vi "Shooter Controller.vi"(8 "error in":errorcluster) -> ()   [LabVIEW 2019]
uses:
  <vilib>/Rock Robotics/WPI/Framework/Completion Status.ctl
  Shooter Setpoints.ctl
  Shooter Operations.ctl
  <vilib>/Rock Robotics/WPI/ThirdParty/REV Robotics/SPARK MAX/Typedef/Spark MAX Idle Mode.ctl
  <vilib>/Rock Robotics/WPI/ThirdParty/REV Robotics/SPARK MAX/Typedef/Spark MAX Control Type.ctl
  <vilib>/Rock Robotics/Network Tables/NT Write Number.vi
  <vilib>/Rock Robotics/Network Tables/NT Read Number.vi
  Framework/Robot Global Data.vi
  28b4446c-53d7-42fe-a716-59488cbe5fc2.vi
  <vilib>/Rock Robotics/Network Tables/NT Write Boolean.vi
panel:
  in  "Flang Setpoint 2":dbl=0.5
  in  "Transfer Setpoint 2":dbl=0.3
  out "shooter 2":dbl(graph)
  out "Waveform Chart 2":dbl(graph)
  out "Waveform Chart":dbl(graph)
  in  "Transfer Setpoint":dbl=0.3
  out "shooter":dbl(graph)
  in  "Flang Setpoint":dbl=0.5
  in  "override":bool=TRUE
  in  "Manual Flywheel":dbl(slide)
  in  "Current Limit A (100)":sgl=100.0
  in  "turret pid":T1={"P Gain"=0.07, "I Gain"=0.0002, "D Gain"=0.0, "F Gain"=0.0, "I Zone"=2.0, "Min Output"=-1.0, "Max Output"=1.0}
  in  "hood pid":T1={"P Gain"=0.1, "I Gain"=0.0002, "D Gain"=0.0, "F Gain"=0.0, "I Zone"=2.0, "Min Output"=-1.0, "Max Output"=1.0}
  in  "flywheel pid":T1={"P Gain"=0.001, "I Gain"=0.0, "D Gain"=0.0, "F Gain"=0.000185, "I Zone"=100.0, "Min Output"=0.0, "Max Output"=1.0}
  in  "Interactive Values":T2
  out "Current\nCmd":string
  in  "Buttons":cluster{"Execute Cmd":bool, "Abort Cmd":bool}
  out "Command Timing":cluster{"Start Time (ms)":u32, "Iterations":i32}
  out "Status":T4
  # "Tip: It may be helpful to observe inputs and sensor values.\nYou may also want to display tuning or debugging controls."
  # "Interactive Command: You may fill in the settings for a command\nand schedule it with the Execute button. You can observe and abort\nany command while fine tuning the code for the controller."
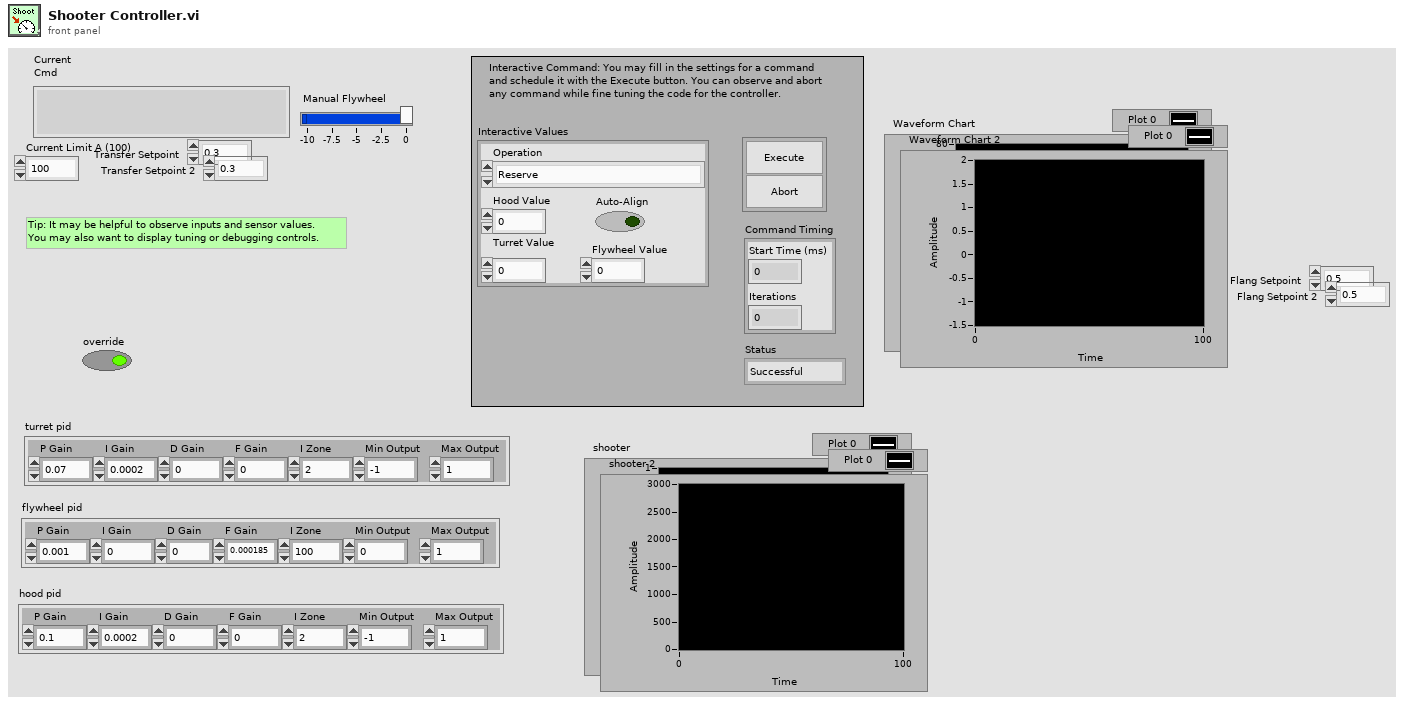
[diagram p1: front panel]
types:
  T1 = cluster{"P Gain":dbl, "I Gain":dbl, "D Gain":dbl, "F Gain":dbl, "I Zone":dbl, "Min Output":dbl, "Max Output":dbl}
  T2 = typedef "Shooter Setpoints.ctl" = cluster{"Operation":T3, "Hood Value":dbl, "Flywheel Value":dbl, "Turret Value":dbl, "Auto-Align":bool}
  T3 = typedef "Shooter Operations.ctl" = enum16{"Reserve", "Read Current", "Immediate", "Shoot", "Reverse Flywheel", "Shoot until no balls"}
  T4 = typedef "Completion Status.ctl" = enum16{"Successful", "Aborted", "Incomplete"}
  T5 = typedef "Spark MAX Idle Mode.ctl" = enum16{"Coast", "Brake"}
  T6 = typedef "WPI_MotorControlDeviceRef.ctl" = cluster{"DeviceStatus":errorcluster, "Type":T7, "PWM":cluster{"PWM Channel":T8, "DeadBand":T9}, "CAN":cluster{"Device Number":u8, "SetOutput VI Ref":variant, "GetOutput VI Ref":variant, "Enable VI Ref":variant, "Disable VI Ref":variant, "Data":variant}, "Invert":bool, "DIO PWM":cluster{"PWM \"Enable\" Channel":T8, "DIOChannel":T10, "PWM Rate":dbl}}
  T7 = typedef "WPI_MotorControlType.ctl" = enum16{"PWM", "CAN", "DIO PWM"}
  T8 = typedef "FPGA_DIOPWMChannel.ctl" = enum8{"PWM 0", "PWM 1", "PWM 2", "PWM 3", "PWM 4", "PWM 5", "PWM 6", "PWM 7", "PWM 8", "PWM 9", "PWM MXP 0", "PWM MXP 1", "PWM MXP 2", "PWM MXP 3", "PWM MXP 4", "PWM MXP 5", "PWM MXP 6", "PWM MXP 7", "PWM MXP 8", "PWM MXP 9", "Invalid"}
  T9 = typedef "WPI_PWMDeadband.ctl" = cluster{"Name":string, "maxPositivePwm":i32, "minPositivePwm":i32, "centerPwm":i32, "maxNegativePwm":i32, "minNegativePwm":i32, "angularRange":u16}
  T10 = typedef "FPGA_DIOChannel.ctl" = enum8{"DIO 0", "DIO 1", "DIO 2", "DIO 3", "DIO 4", "DIO 5", "DIO 6", "DIO 7", "DIO 8", "DIO 9", "DIO MXP 0", "DIO MXP 1", "DIO MXP 2", "DIO MXP 3", "DIO MXP 4", "DIO MXP 5", "DIO MXP 6", "DIO MXP 7", "DIO MXP 8", "DIO MXP 9", "DIO MXP 10", "DIO MXP 11", "DIO MXP 12", "DIO MXP 13", "DIO MXP 14", "DIO MXP 15", "SPI Port CS1", "SPI Port CS2", "SPI Port CS3", "SPI Port MISO", "SPI Port MOSI", "Invalid"}
  T11 = typedef "Command Status Info.ctl" = cluster{"Name":string, "Status":T4, "notifier out":T12}
  T12 = typedef "Completion Notifier.ctl" = refnum<notifier>
  T13 = cluster{"Current Command":T2, "Command Timing":cluster{"Start Time (ms)":u32, "Iterations":i32}, "Command Arguments":cluster{"Command Info":T11, "Description":string, "Default Command":T2, "queue out":refnum<queue>, "Subsystem Name":string}}
  T14 = typedef "Spark MAX Control Type.ctl" = enum16{"Percent VBus", "Voltage", "Velocity", "Position", "Smart Motion", "Current", "Smart Velocity"}
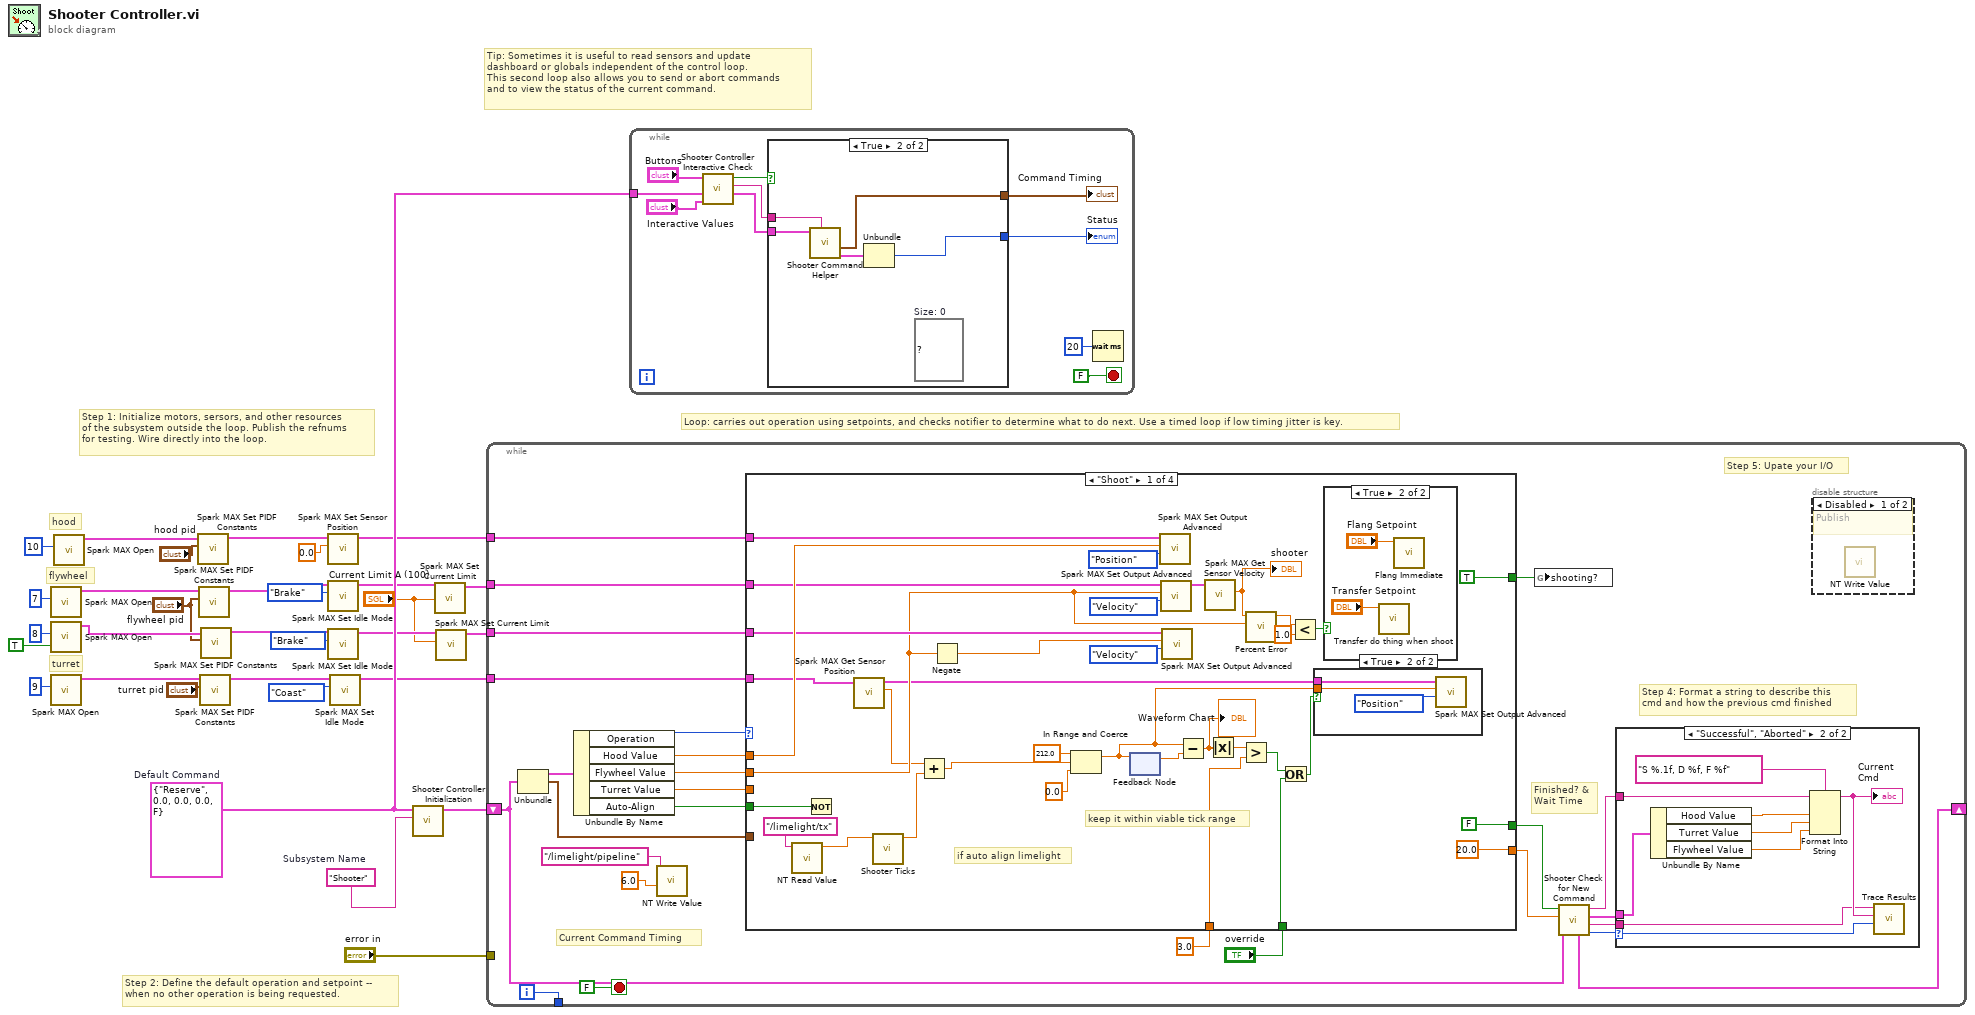
[diagram p0: block diagram]
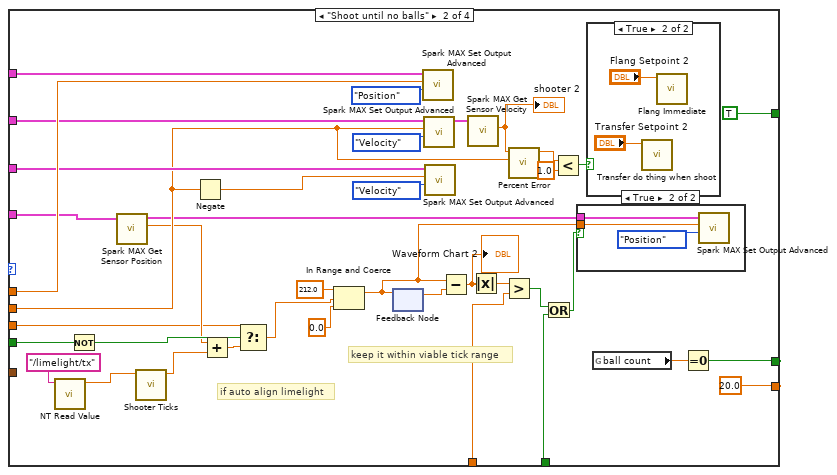
[diagram p6: hidden frame]
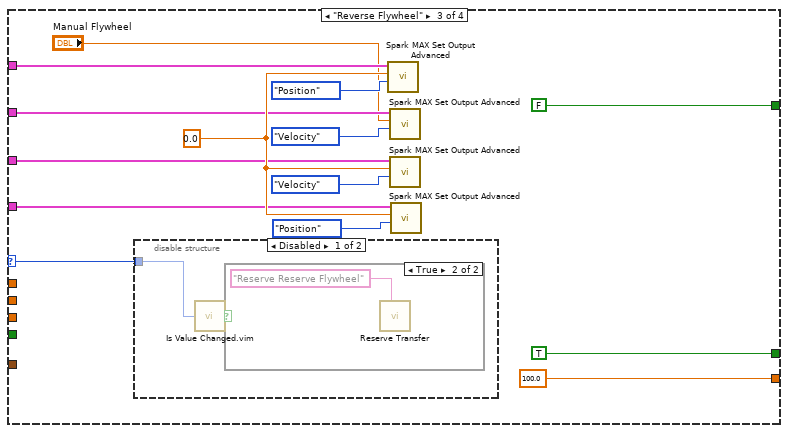
[diagram p9: hidden frame]
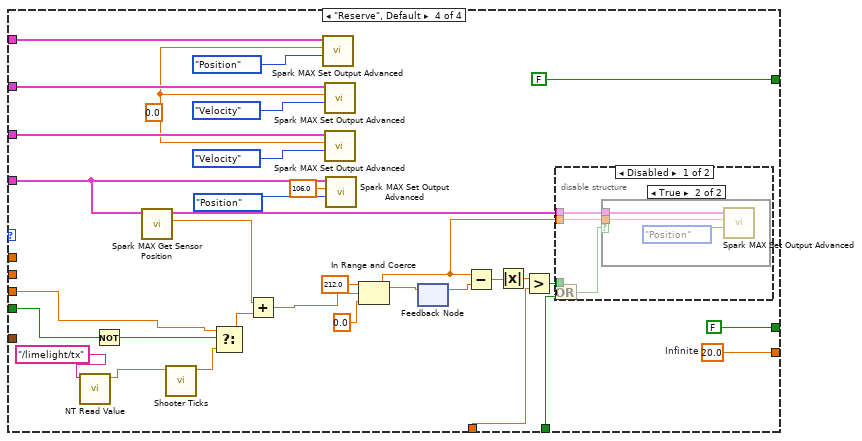
[diagram p12: hidden frame]
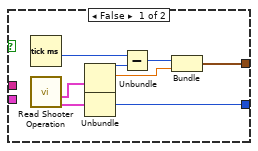
[diagram p15: hidden frame]
diagram:
  w28 = T2 {"Operation"=enum."Reserve", "Hood Value"=0.0, "Flywheel Value"=0.0, "Turret Value"=0.0, "Auto-Align"=FALSE}  # Default Command
  w29 = "Shooter"  # Subsystem Name
  # "turret"
  # "flywheel"
  # "hood"
  # "Tip: Sometimes it is useful to read sensors and update\ndashboard or globals independent of the control loop.\nThis second loop also allows you to send or abort commands\nand to view the status of the current command."
  # "Step 2: Define the default operation and setpoint --\nwhen no other operation is being requested."
  # "Step 1: Initialize motors, sersors, and other resources\nof the subsystem outside the loop. Publish the refnums\nfor testing. Wire directly into the loop."
  # "Loop: carries out operation using setpoints, and checks notifier to determine what to do next. Use a timed loop if low timing jitter is key."
  n1 = call <vilib>:"Spark MAX Open.vi"("Device Number"=u8 7) -> ("MotorControlDeviceRef"=w16:T6)  [unwired: 9 in, 1 out]
  n2 = call <vilib>:"Spark MAX Open.vi"("Invert"=TRUE, "Device Number"=u8 8) -> ("MotorControlDeviceRef"=w15:T6)  [unwired: 8 in, 1 out]
  n3 = call <vilib>:"Spark MAX Open.vi"("Device Number"=u8 9) -> ("MotorControlDeviceRef"=w14:T6)  [unwired: 9 in, 1 out]
  n4 = call <vilib>:"Spark MAX Open.vi"("Device Number"=u8 10) -> ("MotorControlDeviceRef"=w21:T6)  [unwired: 9 in, 1 out]
  n5 = call <vilib>:"Spark MAX Set PIDF Constants.vi"("PID Constants"="hood pid", "MotorControlDeviceRef"=w21) -> ("MotorControlDeviceRef"=w20:T6)  [unwired: 8 in, 1 out]
  n6 = call <vilib>:"Spark MAX Set PIDF Constants.vi"("PID Constants"="flywheel pid", "MotorControlDeviceRef"=w16) -> ("MotorControlDeviceRef"=w11:T6)  [unwired: 8 in, 1 out]
  n7 = call <vilib>:"Spark MAX Set PIDF Constants.vi"("PID Constants"="turret pid", "MotorControlDeviceRef"=w14) -> ("MotorControlDeviceRef"=w8:T6)  [unwired: 8 in, 1 out]
  n8 = call <vilib>:"Spark MAX Set PIDF Constants.vi"("PID Constants"="flywheel pid", "MotorControlDeviceRef"=w15) -> ("MotorControlDeviceRef"=w12:T6)  [unwired: 8 in, 1 out]
  n9 = call <vilib>:"Spark MAX Set Sensor Position.vi"("Position"=0.0, "MotorControlDeviceRef"=w20) -> ("MotorControlDeviceRef"=w18:T6)  [unwired: 8 in, 1 out]
  n10 = call <vilib>:"Spark MAX Set Idle Mode.vi"("Idle Mode"=Spark_MAX_Idle_Mode."Brake", "MotorControlDeviceRef in"=w11) -> ("MotorControlDeviceRef out"=w6:T6)  [unwired: 8 in, 1 out]
  n11 = call <vilib>:"Spark MAX Set Idle Mode.vi"("Idle Mode"=Spark_MAX_Idle_Mode."Brake", "MotorControlDeviceRef in"=w12) -> ("MotorControlDeviceRef out"=w4:T6)  [unwired: 8 in, 1 out]
  n12 = call <vilib>:"Spark MAX Set Idle Mode.vi"("Idle Mode"=Spark_MAX_Idle_Mode."Coast", "MotorControlDeviceRef in"=w8) -> ("MotorControlDeviceRef out"=w1:T6)  [unwired: 8 in, 1 out]
  n13 = call "Shooter Controller Initialization.vi"("Subsystem Name"=w29, "Default Command"=w28) -> ("Current Command"=w30:T13)  [unwired: 9 in]
  n14 = call <vilib>:"Spark MAX Set Current Limit.vi"("Current Limit A (100)"="Current Limit A (100)", "MotorControlDeviceRef in"=w6) -> ("MotorControlDeviceRef out"=w5:T6)  [unwired: 8 in, 1 out]
  n15 = call <vilib>:"Spark MAX Set Current Limit.vi"("Current Limit A (100)"="Current Limit A (100)", "MotorControlDeviceRef in"=w4) -> ("MotorControlDeviceRef out"=w3:T6)  [unwired: 8 in, 1 out]
  n16 = while {
    shift-right: [w53] -> _
    shift-left: w30 -> [w46]
    tunnel: [w56] -> _
    tunnel: "error in" -> [_]
    tunnel: w18 -> [w45]
    tunnel: w5 -> [w44]
    tunnel: w1 -> [w43]
    tunnel: w3 -> [w39]
    i -> [w56]
    stop <- FALSE stop-if-true
    # "Step 5: Upate your I/O"
    # "Step 4: Format a string to describe this\ncmd and how the previous cmd finished"
    # "Current Command Timing"
    # "Finished? &\nWait Time"
    n17 = Unbundle(w46) -> ("Current Command"=w55:T2, "Command Timing"=w54:cluster{"Start Time (ms)":u32, "Iterations":i32})  [unwired: 1 out]
    n18 = Unbundle By Name(w55) -> ("Operation"=w37:T3, "Hood Value"=w40:dbl, "Flywheel Value"=w42:dbl, "Turret Value"=w41:dbl, "Auto-Align"=w32:bool)
    n19 = call-poly <vilib>:"NT Write Value.vi"("Numeric"=6.0, "Name"="/limelight/pipeline") -> ()  [unwired: 9 in, 1 out]
    n20 = case shown="\"Shoot\"" w37 {
      selector: w37 -> [_ _ w151 _]
      tunnel: [20.0 ("Infinite") 20.0 ("Infinite") 100.0 ("Infinite") w199] -> w51
      tunnel: [FALSE ("ignore previous (F)") w111 TRUE ("ignore previous (F)") FALSE ("ignore previous (F)")] -> w52
      tunnel: w54 -> [_ _ _ _]
      tunnel: w45 -> [w99 w144 w159 w196]
      tunnel: w44 -> [w88 w132 w158 w193]
      tunnel: w43 -> [w81 w125 w156 w186]
      tunnel: w40 -> [w98 w143 _ _]
      tunnel: w42 -> [w85 w129 _ _]
      tunnel: w41 -> [_ w108 _ w183]
      tunnel: w32 -> [w97 w142 _ w185]
      tunnel: w39 -> [w87 w131 w157 w191]
      tunnel: [TRUE ("shooting?") TRUE ("shooting?") FALSE ("shooting?") FALSE ("shooting?")] -> w38
      tunnel: "override" -> [w72 w116 _ w172]
      tunnel: 3.0 ("y") -> [w71 w115 _ w174]
      frame "Shoot" {
        # "keep it within viable tick range"
        # "if auto align limelight"
        n21 = call-poly <vilib>:"NT Read Value.vi"("Name"="/limelight/tx") -> ("Numeric"=w69:dbl)  [unwired: 9 in, 1 out]
        n22 = Not(x=w97) -> ()  [unwired: 1 out]
        n23 = call <vilib>:"Spark MAX Get Sensor Position.vi"("MotorControlDevRef in"=w81) -> ("Sensor Position"=w79:dbl, "MotorControlDevRef out"=w80:T6)  [unwired: 7 in, 2 out]
        n24 = call "Shooter Ticks.vi"("limelight"=w69) -> ("ticks"=w68:dbl)  [unwired: 10 in]
        n25 = Add(x=w79, y=w68) -> (x+y=w67:dbl)
        n26 = Negate(x=w85) -> (-x=w90:dbl)
        n27 = In Range and Coerce(upper limit=212.0, x=w67, lower limit=0.0) -> (coerced(x)=w76:dbl)  [unwired: 1 out]
        n28 = feedback-in #1(w76) -> ()
        n29 = feedback #1() -> (w78:dbl)  [unwired: 1 in]
        n30 = call <vilib>:"Spark MAX Set Output Advanced.vi"("Control Mode"=Spark_MAX_Control_Type."Position", "Setpoint"=w98, "MotorControlDevRef"=w99) -> ()  [unwired: 7 in, 2 out]
        n31 = call <vilib>:"Spark MAX Set Output Advanced.vi"("Control Mode"=Spark_MAX_Control_Type."Velocity", "Setpoint"=w85, "MotorControlDevRef"=w88) -> ("MotorControlDevRef"=w86:T6)  [unwired: 7 in, 1 out]
        n32 = call <vilib>:"Spark MAX Set Output Advanced.vi"("Control Mode"=Spark_MAX_Control_Type."Velocity", "Setpoint"=w90, "MotorControlDevRef"=w87) -> ()  [unwired: 7 in, 2 out]
        n33 = Subtract(x=w76, y=w78) -> (x-y=w70:dbl)
        "Waveform Chart" <- w70
        n34 = call <vilib>:"Spark MAX Get Sensor Velocity.vi"("MotorControlDevRef in"=w86) -> ("Sensor Velocity"=w73:dbl)  [unwired: 7 in, 3 out]
        "shooter" <- w73
        n35 = Absolute Value(x=w70) -> (abs(x)=w77:dbl)
        n36 = Greater?(x=w77, y=w71) -> (0:w75:bool)
        n37 = call "Percent Error.vi"("Expected"=w85, "Observed"=w73) -> ("Percent Error"=w84:dbl)  [unwired: 9 in]
        n38 = Or(x=w75, y=w72) -> (x .or. y?=w74:bool)
        n39 = Less?(x=w84, y=1.0) -> (x < y?=w82:bool)
        n40 = case shown="True" w74 {
          tunnel: w80 -> [_ w104]
          tunnel: w76 -> [_ w102]
          frame False {
          }
          frame True {
            n41 = call <vilib>:"Spark MAX Set Output Advanced.vi"("Control Mode"=Spark_MAX_Control_Type."Position", "Setpoint"=w102, "MotorControlDevRef"=w104) -> ()  [unwired: 7 in, 2 out]
          }
        }
        n42 = case shown="True" w82 {
          frame False {
          }
          frame True {
            n43 = call "Transfer do thing when shoot.vi"("Setpoint"="Transfer Setpoint") -> ()  [unwired: 10 in, 1 out]
            n44 = call "Flang Immediate.vi"("Setpoint"="Flang Setpoint") -> ()  [unwired: 10 in, 1 out]
          }
        }
      }
      frame "Shoot until no balls" {
        # "keep it within viable tick range"
        # "if auto align limelight"
        n45 = call-poly <vilib>:"NT Read Value.vi"("Name"="/limelight/tx") -> ("Numeric"=w113:dbl)  [unwired: 9 in, 1 out]
        n46 = Not(x=w142) -> (.not. x?=w141:bool)
        n47 = call <vilib>:"Spark MAX Get Sensor Position.vi"("MotorControlDevRef in"=w125) -> ("Sensor Position"=w123:dbl, "MotorControlDevRef out"=w124:T6)  [unwired: 7 in, 2 out]
        n48 = call "Shooter Ticks.vi"("limelight"=w113) -> ("ticks"=w110:dbl)  [unwired: 10 in]
        n49 = Negate(x=w129) -> (-x=w134:dbl)
        n50 = Add(x=w123, y=w110) -> (x+y=w109:dbl)
        n51 = Select(t=w108, s=w141, f=w109) -> (s? t:f=w107:dbl)
        n52 = In Range and Coerce(upper limit=212.0, x=w107, lower limit=0.0) -> (coerced(x)=w120:dbl)  [unwired: 1 out]
        n53 = feedback-in #2(w120) -> ()
        n54 = feedback #2() -> (w122:dbl)  [unwired: 1 in]
        n55 = call <vilib>:"Spark MAX Set Output Advanced.vi"("Control Mode"=Spark_MAX_Control_Type."Position", "Setpoint"=w143, "MotorControlDevRef"=w144) -> ()  [unwired: 7 in, 2 out]
        n56 = call <vilib>:"Spark MAX Set Output Advanced.vi"("Control Mode"=Spark_MAX_Control_Type."Velocity", "Setpoint"=w129, "MotorControlDevRef"=w132) -> ("MotorControlDevRef"=w130:T6)  [unwired: 7 in, 1 out]
        n57 = call <vilib>:"Spark MAX Set Output Advanced.vi"("Control Mode"=Spark_MAX_Control_Type."Velocity", "Setpoint"=w134, "MotorControlDevRef"=w131) -> ()  [unwired: 7 in, 2 out]
        n58 = Subtract(x=w120, y=w122) -> (x-y=w114:dbl)
        "Waveform Chart 2" <- w114
        n59 = call <vilib>:"Spark MAX Get Sensor Velocity.vi"("MotorControlDevRef in"=w130) -> ("Sensor Velocity"=w117:dbl)  [unwired: 7 in, 3 out]
        "shooter 2" <- w117
        n60 = Absolute Value(x=w114) -> (abs(x)=w121:dbl)
        n61 = Greater?(x=w121, y=w115) -> (0:w119:bool)
        n62 = call "Percent Error.vi"("Expected"=w129, "Observed"=w117) -> ("Percent Error"=w128:dbl)  [unwired: 9 in]
        n63 = Or(x=w119, y=w116) -> (x .or. y?=w118:bool)
        n64 = Less?(x=w128, y=1.0) -> (x < y?=w126:bool)
        n65 = case shown="True" w118 {
          tunnel: w124 -> [_ w148]
          tunnel: w120 -> [_ w146]
          frame False {
          }
          frame True {
            n66 = call <vilib>:"Spark MAX Set Output Advanced.vi"("Control Mode"=Spark_MAX_Control_Type."Position", "Setpoint"=w146, "MotorControlDevRef"=w148) -> ()  [unwired: 7 in, 2 out]
          }
        }
        n67 = case shown="True" w126 {
          frame False {
          }
          frame True {
            n68 = call "Transfer do thing when shoot.vi"("Setpoint"="Transfer Setpoint 2") -> ()  [unwired: 10 in, 1 out]
            n69 = call "Flang Immediate.vi"("Setpoint"="Flang Setpoint 2") -> ()  [unwired: 10 in, 1 out]
          }
        }
        n70 = global read "Robot Global Data.vi" "ball count"() -> (w112:dbl)
        n71 = Equal To 0?(x=w112) -> (x = 0?=w111:bool)
      }
      frame "Reverse Flywheel" {
        w163 = 0.0 ("Setpoint")
        n72 = disable-structure shown="Disabled" {
          disable-tunnel: w151 -> [w165 _]
          frame Disabled {
            n73 = call "Is Value Changed.vim"("value"=w165) -> ("changed or first call?"=w166:bool)
            n74 = case shown="True" w166 {
              frame False {
              }
              frame True {
                n75 = call "Reserve Transfer.vi"("Description"="Reserve Reserve Flywheel") -> ()  [unwired: 10 in, 1 out]
              }
            }
          }
          frame Enabled {
          }
        }
        n76 = call <vilib>:"Spark MAX Set Output Advanced.vi"("Control Mode"=Spark_MAX_Control_Type."Position", "Setpoint"=w163, "MotorControlDevRef"=w159) -> ()  [unwired: 7 in, 2 out]
        n77 = call <vilib>:"Spark MAX Set Output Advanced.vi"("Control Mode"=Spark_MAX_Control_Type."Velocity", "Setpoint"="Manual Flywheel", "MotorControlDevRef"=w158) -> ()  [unwired: 7 in, 2 out]
        n78 = call <vilib>:"Spark MAX Set Output Advanced.vi"("Control Mode"=Spark_MAX_Control_Type."Velocity", "Setpoint"=w163, "MotorControlDevRef"=w157) -> ()  [unwired: 7 in, 2 out]
        n79 = call <vilib>:"Spark MAX Set Output Advanced.vi"("Control Mode"=Spark_MAX_Control_Type."Position", "Setpoint"=w163, "MotorControlDevRef"=w156) -> ()  [unwired: 7 in, 2 out]
      }
      frame "Reserve", Default {
        w190 = 0.0 ("Setpoint")
        w199 = 20.0  # Infinite
        n80 = call-poly <vilib>:"NT Read Value.vi"("Name"="/limelight/tx") -> ("Numeric"=w169:dbl)  [unwired: 9 in, 1 out]
        n81 = Not(x=w185) -> (.not. x?=w184:bool)
        n82 = call <vilib>:"Spark MAX Get Sensor Position.vi"("MotorControlDevRef in"=w186) -> ("Sensor Position"=w179:dbl, "MotorControlDevRef out"=w188:T6)  [unwired: 7 in, 2 out]
        n83 = call "Shooter Ticks.vi"("limelight"=w169) -> ("ticks"=w182:dbl)  [unwired: 10 in]
        n84 = Select(t=w183, s=w184, f=w182) -> (s? t:f=w181:dbl)
        n85 = Add(x=w179, y=w181) -> (x+y=w180:dbl)
        n86 = call <vilib>:"Spark MAX Set Output Advanced.vi"("Control Mode"=Spark_MAX_Control_Type."Position", "Setpoint"=w190, "MotorControlDevRef"=w196) -> ()  [unwired: 7 in, 2 out]
        n87 = call <vilib>:"Spark MAX Set Output Advanced.vi"("Control Mode"=Spark_MAX_Control_Type."Velocity", "Setpoint"=w190, "MotorControlDevRef"=w193) -> ()  [unwired: 7 in, 2 out]
        n88 = call <vilib>:"Spark MAX Set Output Advanced.vi"("Control Mode"=Spark_MAX_Control_Type."Velocity", "Setpoint"=w190, "MotorControlDevRef"=w191) -> ()  [unwired: 7 in, 2 out]
        n89 = call <vilib>:"Spark MAX Set Output Advanced.vi"("Control Mode"=Spark_MAX_Control_Type."Position", "Setpoint"=106.0, "MotorControlDevRef"=w186) -> ()  [unwired: 7 in, 2 out]
        n90 = In Range and Coerce(upper limit=212.0, x=w180, lower limit=0.0) -> (coerced(x)=w177:dbl)  [unwired: 1 out]
        n91 = feedback #3() -> (w178:dbl)  [unwired: 1 in]
        n92 = feedback-in #3(w177) -> ()
        n93 = Subtract(x=w177, y=w178) -> (x-y=w176:dbl)
        n94 = Absolute Value(x=w176) -> (abs(x)=w175:dbl)
        n95 = Greater?(x=w175, y=w174) -> (0:w173:bool)
        n96 = disable-structure shown="Disabled" {
          disable-tunnel: w188 -> [w204 _]
          disable-tunnel: w177 -> [w203 _]
          disable-tunnel: w173 -> [w202 _]
          disable-tunnel: w172 -> [w201 _]
          frame Disabled {
            n97 = Or(x=w202, y=w201) -> (x .or. y?=w200:bool)
            n98 = case shown="True" w200 {
              tunnel: w204 -> [_ w207]
              tunnel: w203 -> [_ w205]
              frame False {
              }
              frame True {
                n99 = call <vilib>:"Spark MAX Set Output Advanced.vi"("Control Mode"=Spark_MAX_Control_Type."Position", "Setpoint"=w205, "MotorControlDevRef"=w207) -> ()  [unwired: 7 in, 2 out]
              }
            }
          }
          frame Enabled {
          }
        }
      }
    }
    n100 = global write "Robot Global Data.vi" "shooting?"(w38) -> ()
    n101 = call "Shooter Check for New Command.vi"("Current Command"=w46, "Wait time (ms)"=w51, "Finished?"=w52) -> ("Completion"=w47:T4, "Subsystem Name"=w48:string, "Current Command"=w49:T2, "Initial Trace String"=w50:string, "NextCommand"=w53:T13)  [unwired: 4 in]
    n102 = case shown="\"Successful\", \"Aborted\"" w47 {
      selector: w47 -> [_ w66]
      tunnel: w50 -> [_ w62]
      tunnel: w49 -> [_ w63]
      tunnel: w48 -> [_ w59]
      frame "Incomplete", Default {
        # "Continuing current command"
      }
      frame "Successful", "Aborted" {
        # "Report and setup for next command"
        n103 = Unbundle By Name(w63) -> ("Hood Value"=w65:dbl, "Turret Value"=w60:dbl, "Flywheel Value"=w58:dbl)
        n104 = Format Into String(format string="S %.1f, D %f, F %f", initial string=w62, w65, w60, w58) -> (resulting string=w61:string)  [unwired: 1 in, 1 out]
        "Current\nCmd" <- w61
        n105 = call <vilib>:"Trace Results.vi"("Status of previous command"=w66, "Description"=w61, "Subsystem"=w59) -> ()  [unwired: 9 in]
      }
    }
    n106 = disable-structure shown="Disabled" {
      frame Disabled {
        # "Publish"
        n107 = call-poly <vilib>:"NT Write Value.vi"() -> ()  [unwired: 11 in, 1 out]
      }
      frame Enabled {
      }
    }
  }
  n108 = while {
    tunnel: w28 -> [w214]
    stop <- FALSE stop-if-true
    n109 = call "Shooter Controller Interactive Check.vi"("Interactive Command in"="Interactive Values", "Default Command"=w214, "Buttons"="Buttons") -> ("Interactive Command out"=w211:T2, "Trace String"=w212:string, "Schedule"=w213:bool)  [unwired: 6 in]
    n110 = case shown="True" w213 {
      tunnel: [w225 w230] -> w210
      tunnel: w211 -> [_ w228]
      tunnel: [w221 w226] -> w209
      tunnel: w212 -> [_ w229]
      frame False {
        n111 = Tick Count (ms)() -> (millisecond timer value=w220:u32)
        n112 = call "Read Shooter Operation.vi"() -> ("Command Info"=w218:T11, "SubSystem Data"=w219:T2)  [unwired: 9 in, 1 out]
        n113 = Unbundle(w219) -> ("Operation"=w224:T3, "Hood Value"=w222:dbl)  [unwired: 3 out]
        n114 = Unbundle(w218) -> ("Status"=w225:T4)  [unwired: 2 out]
        n115 = Subtract(x=w220, y=w224) -> (x-y=w223:u32)
        n116 = Bundle(w223, "Hood Value"=w222) -> (w221:cluster{u32, "Hood Value":dbl})  [unwired: 1 in]
      }
      frame True {
        (unwired) map{string, i32} {}  # Size: 0
        n117 = call "Shooter Command Helper.vi"("Description"=w229, "SubSystem Data"=w228) -> ("Command Info Out"=w227:T11, "Command Timing"=w226:cluster{"Start Time (ms)":u32, "Iterations":i32})  [unwired: 7 in, 1 out]
        n118 = Unbundle(w227) -> ("Status"=w230:T4)  [unwired: 2 out]
      }
    }
    "Status" <- w210
    "Command Timing" <- w209
    n119 = Wait (ms)(milliseconds to wait=u32 20) -> ()  [unwired: 1 out]
  }
